vi "InstrumentNames.vi"(8 "error in (no error)":errorcluster, 11 "Instrument type":T1(ring)) -> (0 "error out":errorcluster, 3 "Instrument names":string[](array[string]))   [LabVIEW 2019, in "InstrControl.lvclass"]
uses:
  InstrControl.lvclass
  InstrumentSetup.vi
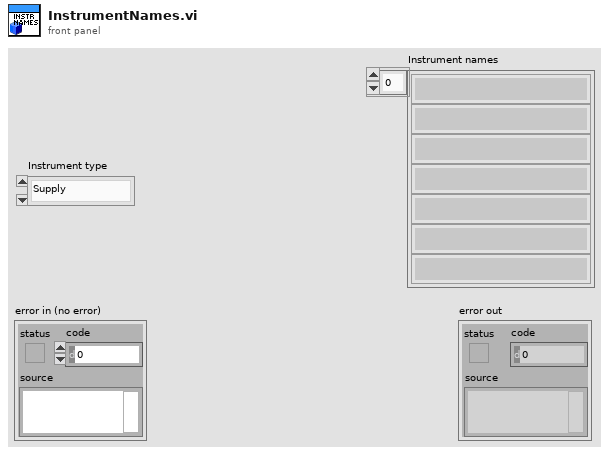
[diagram p1: front panel]
types:
  T1 = enum16{"Supply", "LCR", "Multimeter", "Switching"}
  T2 = cluster{"KE 2410":cluster{"Instrument name":string, "GPIB address":string, "Instrument type":u16}, "KE 6517":cluster{"Instrument name":string, "GPIB address":string, "Instrument type":u16}, "KE 487":cluster{"Instrument name":string, "GPIB address":string, "Instrument type":u16}, "KE 236":cluster{"Instrument name":string, "GPIB address":string, "Instrument type":u16}, "KE 487_2":cluster{"Instrument name":string, "GPIB address":string, "Instrument type":u16}, "WK 6440B":cluster{"Instrument name":string, "GPIB address":string, "Instrument type":u16}, "WK 6425":cluster{"Instrument name":string, "GPIB address":string, "Instrument type":u16}, "Pickering Matrix":cluster{"Instrument name":string, "GPIB address":string, "Instrument type":u16}, "KE 2000":cluster{"Instrument name":string, "GPIB address":string, "Instrument type":u16}, "KE3706A Switching":cluster{"Instrument name":string, "GPIB address":string, "Instrument type":u16}}
  T3 = cluster{"Instrument name":string, "GPIB address":string, "Instrument type":u16}[]
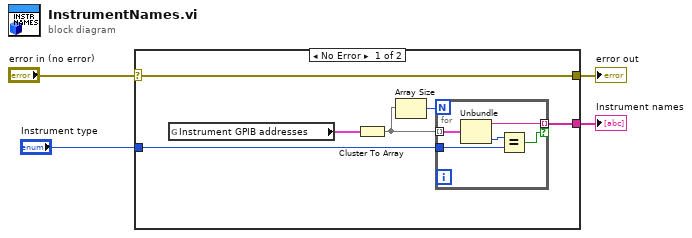
[diagram p0: block diagram]
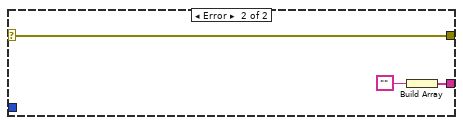
[diagram p2: hidden frame]
diagram:
  n1 = case shown="No Error" "error in (no error)" {
    selector: "error in (no error)" -> [w10 w18]
    tunnel: [w10 w18] -> w3
    tunnel: "Instrument type" -> [w6 _]
    tunnel: [w5 w16] -> w1
    frame No Error {
      n2 = global read "InstrumentSetup.vi" "Instrument GPIB addresses"() -> (w9:T2)
      n3 = Cluster To Array(cluster=w9) -> (array=w7:T3)
      n4 = Array Size(array=w7) -> (size(s)=w8:i32)
      n5 = for {
        N: w8 -> [_]
        tunnel: w7 -> [w15] mode=indexing
        tunnel: w6 -> [w13]
        tunnel: [w11] -> w5 mode=indexing if=w12
        n6 = Unbundle(w15) -> ("Instrument name"=w11:string, "Instrument type"=w14:u16)  [unwired: 1 out]
        n7 = Equal?(x=w14, y=w13) -> (x = y?=w12:bool)
      }
    }
    frame Error {
      n8 = Build Array("") -> (w16:string[])
    }
  }
  "error out" <- w3
  "Instrument names" <- w1
